vi "TDMS_View.vi"() -> ()   [LabVIEW 2011]
doc: "打开TDMS文件查看器"
panel:
  in  "file path":path caption="文件路径"
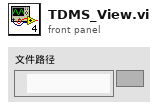
[diagram p1: front panel]
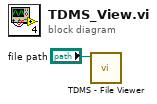
[diagram p0: block diagram]
diagram:
  n1 = call <vilib>:"TDMS - File Viewer.vi"("file path"="file path") -> ()  [unwired: 5 in, 2 out]
